vi "AH_PreCMD.vi"(8 "error in (no error)":errorcluster, 9 "CMD":string, 10 "Data Cluster In":T1 {"GUI Data Cluster"."SBR" format="%08b"}, 11 "Config Cluster In":T3={"General"={"Config.ini"=path "", "Default Logging Path"=path ""}, "Hardware"={"AHC VISA COM"="", "Measure Rate (1/s)"=0, "Global T VAR"="", "Global B VAR"="", "Average"=4, "Bias"=0, "Cable"={"Length"=0.0, "Resistance"=0.0, "Inductance"=0.0, "Capacitance"=0.0}, "Tracking"=0, "Voltage"=0.0}, "Operation"={"Operation Mode"=enum."Logging", "Status"="", "NewLog?"=FALSE}}) -> (0 "error IO":errorcluster, 2 "Data Cluster Out":T1 {"GUI Data Cluster"."SBR" format="%08b"}, 3 "Configuration Cluster Out":T3={"General"={"Config.ini"=path "", "Default Logging Path"=path ""}, "Hardware"={"AHC VISA COM"="", "Measure Rate (1/s)"=0, "Global T VAR"="", "Global B VAR"="", "Average"=4, "Bias"=0, "Cable"={"Length"=0.0, "Resistance"=0.0, "Inductance"=0.0, "Capacitance"=0.0}, "Tracking"=0, "Voltage"=0.0}, "Operation"={"Operation Mode"=enum."Idle-Off", "Status"="", "NewLog?"=FALSE}})   [LabVIEW 2021]
uses:
  Config_Cluster.ctl
  Mode_Enum.ctl
  Data_Cluster.ctl
  Measurement_Cluster.ctl
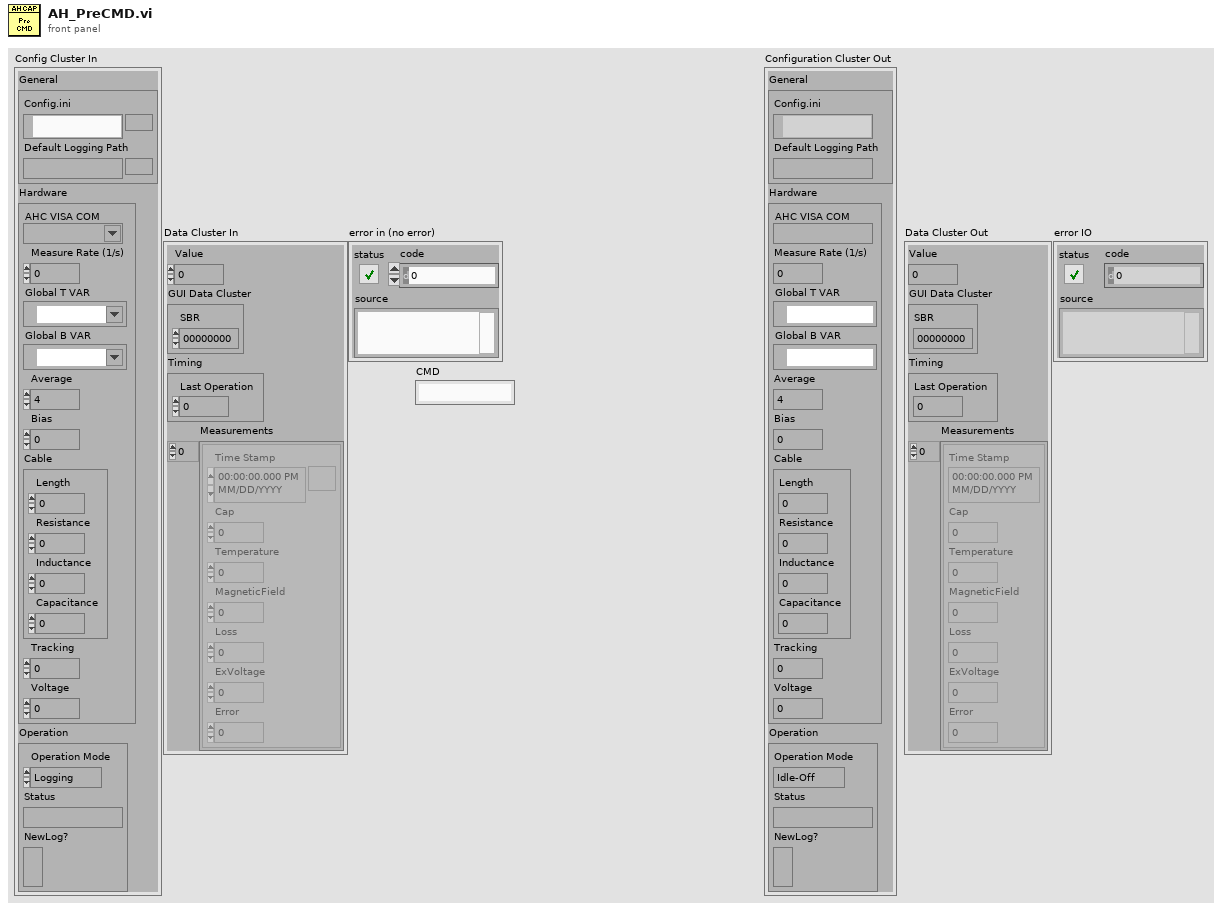
[diagram p1: front panel]
types:
  T1 = typedef "Data_Cluster.ctl" = cluster{"Value":dbl, "GUI Data Cluster":cluster{"SBR":u16}, "Timing":cluster{"Last Operation":dbl}, "Measurements":T2[]}
  T2 = typedef "Measurement_Cluster.ctl" = cluster{"Time Stamp":timestamp, "Cap":dbl, "Temperature":dbl, "MagneticField":dbl, "Loss":dbl, "ExVoltage":dbl, "Error":dbl}
  T3 = typedef "Config_Cluster.ctl" = cluster{"General":cluster{"Config.ini":path, "Default Logging Path":path}, "Hardware":cluster{"AHC VISA COM":refnum<visa-resource-name>, "Measure Rate (1/s)":i32, "Global T VAR":refnum<k21>, "Global B VAR":refnum<k21>, "Average":u8, "Bias":u8, "Cable":cluster{"Length":dbl, "Resistance":dbl, "Inductance":dbl, "Capacitance":dbl}, "Tracking":u8, "Voltage":dbl}, "Operation":cluster{"Operation Mode":T4, "Status":string, "NewLog?":bool}}
  T4 = typedef "Mode_Enum.ctl" = enum16{"Logging", "Idle-Off", "Idle"}
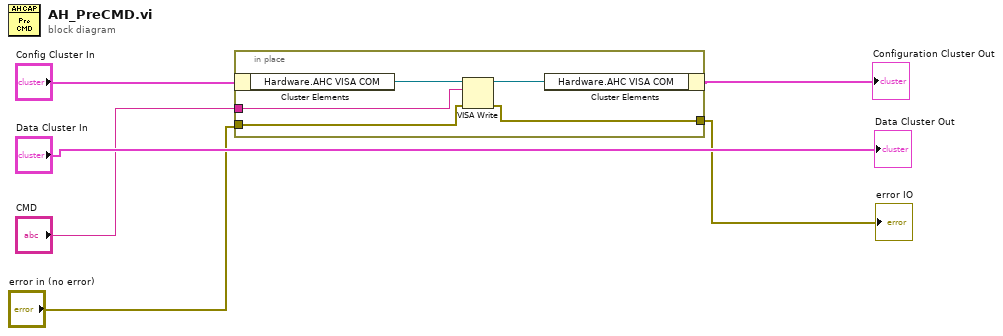
[diagram p0: block diagram]
diagram:
  n1 = in-place {
    in-place-border: "error in (no error)" -> [w9]
    in-place-border: [w8] -> w2
    in-place-border: "CMD" -> [w7]
    n2 = in-place-cluster #1("Config Cluster In") -> ("Hardware.AHC VISA COM"=w11:refnum<visa-resource-name>)
    n3 = VISA Write(VISA resource name=w11, write buffer=w7, error in (no error)=w9) -> (VISA resource name out=w10:refnum<visa-resource-name>, error out=w8:errorcluster)  [unwired: 1 out]
    n4 = in-place-cluster #1("Hardware.AHC VISA COM"=w10) -> (→"Configuration Cluster Out":T3)
  }
  "error IO" <- w2
  "Data Cluster Out" <- "Data Cluster In"
